vi "Waveform_Extract from StartEnd and Duration.vi"(9 "From End(f)\nFrom Beginning(t)":bool, 10 "Duration(S)":dbl, 11 "Raw Data Waveform":T1) -> (1 "End Out":i32, 2 "Start Out":i32, 3 "Raw Data Waveform Out":T1)   [LabVIEW 2020]
uses:
  Universal Controls/Waveform_Data.ctl
  Universal Controls/Read Write Button.ctl
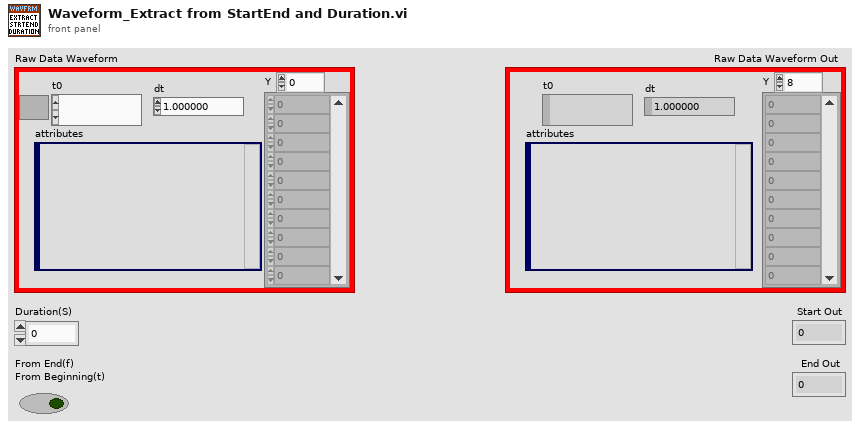
[diagram p1: front panel]
types:
  T1 = typedef "Waveform_Data.ctl" = waveform(dbl)
  T2 = typedef "Read Write Button.ctl" = bool
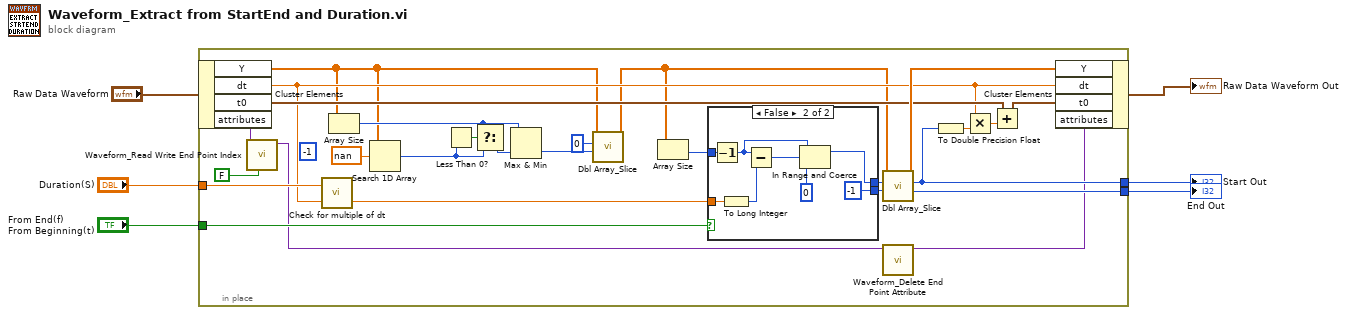
[diagram p0: block diagram]
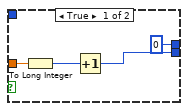
[diagram p2: hidden frame]
diagram:
  n1 = in-place {
    in-place-border: [w21] -> w2
    in-place-border: [w29] -> w3
    in-place-border: "From End(f)\nFrom Beginning(t)" -> [w28]
    in-place-border: "Duration(S)" -> [w27]
    (unwired) -1 ("f")
    n2 = in-place-cluster #1("Raw Data Waveform") -> ("Y"=w9:dbl[], "dt"=w26:dbl, "t0"=w31:timestamp, "attributes"=w11:variant)
    n3 = call "Waveform_Read Write End Point Index.vi"("Read(f)\nWrite(t)"=T2 FALSE ("Read(f)\nWrite(t)"), "Waveform Attributes"=w11) -> ("Waveform Attributes Out"=w10:variant)  [unwired: 6 in, 3 out]
    n4 = call <vilib>:"Check for multiple of dt.vi"("dt"=w26, "time"=w27) -> ("iQuotient"=w25:dbl)  [unwired: 1 out]
    n5 = Array Size(array=w9) -> (size(s)=w18:i32)
    n6 = Search 1D Array(1D array=w9, element=nan) -> (index of element=w7:i32)  [unwired: 1 in]
    n7 = Less Than 0?(x=w7) -> (x < 0?=w20:bool)
    n8 = Select(t=w18, s=w20, f=w7) -> (s? t:f=w19:i32)
    n9 = Max & Min(x=w18, y=w19) -> (min(x,y)=w17:i32)  [unwired: 1 out]
    n10 = call "Dbl Array_Slice.vi"("End Index\n(-1) Last point"=w17, "Start Index"=0, "Array"=w9) -> ("Subarray (array[i:j]) Out"=w14:dbl[])  [unwired: 1 in, 7 out]
    n11 = Array Size(array=w14) -> (size(s)=w15:i32)
    n12 = case shown="False" w28 {
      tunnel: [0 w38] -> w23
      tunnel: w25 -> [w37 w43]
      tunnel: [w34 -1 ("Start")] -> w24
      tunnel: w15 -> [_ w45]
      frame True {
        n13 = To Long Integer(number=w37) -> (32bit integer=w35:i32)
        n14 = Increment(x=w35) -> (x+1=w34:i32)
      }
      frame False {
        n15 = Decrement(x=w45) -> (x-1=w40:i32)
        n16 = To Long Integer(number=w43) -> (32bit integer=w42:i32)
        n17 = Subtract(x=w40, y=w42) -> (x-y=w39:i32)
        n18 = In Range and Coerce(upper limit=w40, x=w39, lower limit=0) -> (coerced(x)=w38:i32)  [unwired: 1 out]
      }
    }
    n19 = call "Dbl Array_Slice.vi"("End Index\n(-1) Last point"=w24, "Start Index"=w23, "Array"=w14) -> ("End Out"=w29:i32, "Start Out"=w21:i32, "Subarray (array[i:j]) Out"=w33:dbl[])  [unwired: 1 in, 5 out]
    n20 = call "Waveform_Delete End Point Attribute.vi"("Waveform Attributes"=w10) -> ("Waveform Attributes Out"=w12:variant)  [unwired: 9 in, 1 out]
    n21 = To Double Precision Float(number=w21) -> (double precision float=w22:dbl)
    n22 = Multiply(x=w26, y=w22) -> (x*y=w32:dbl)
    n23 = Add(x=w31, y=w32) -> (x+y=w30:timestamp)
    n24 = in-place-cluster #1("Y"=w33, "dt"=w26, "t0"=w30, "attributes"=w12) -> (→"Raw Data Waveform Out":T1)
  }
  "End Out" <- w3
  "Start Out" <- w2
